vi "update.vi"(8 "error in (no error)":errorcluster, 10 "adapter executability":T1={"instrument"=TRUE, "trajectory"=TRUE, "scanHead"=TRUE, "DAQ"=TRUE, "imageAssembler"=TRUE, "dataCollection"=TRUE, "display"=TRUE, "analyser"=TRUE, "stimulator"=TRUE}, 11 "ImagingModeDL090130Frame in":refnum<class "ImagingModeDL090130Frame.lvclass">=refnum) -> (0 "error out":errorcluster, 3 "ImagingModeDL090130Frame out":refnum<class "ImagingModeDL090130Frame.lvclass">)   [LabVIEW 2010, in "ImagingModeDL090130Frame.lvclass"]
uses:
  ImagingModeDL090130Frame.lvclass
  ImagingModeDL090923Scaffold/ImagingModeDL090923Scaffold/adapter_executability_cluster.ctl
  ImagingModeDL090923Scaffold/ImagingModeDL090923Scaffold/ImagingModeDL090923Scaffold.lvclass
  ScanHead/GenericScanHead/GenericScanHead/GenericScanHead.lvclass
  ImageAssembler/GenericImageAssembler/GenericImageAssembler/GenericImageAssembler.lvclass
  DataCollection/GenericDataCollection/GenericDataCollection/GenericDataCollection.lvclass
  common/xcontrols/XSettings/XSettings/XSettings.xctl
  common/classes/ErrorController/ErrorController/class_data.vi
  common/classes/ErrorController/ErrorController/ErrorController.lvclass
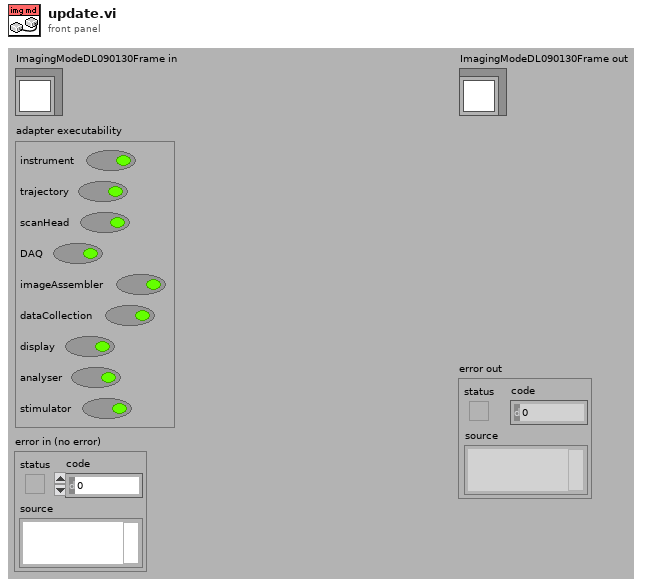
[diagram p1: front panel]
types:
  T1 = typedef "ImagingModeDL090923Scaffold.lvclass/adapter_executability_cluster.ctl" = cluster{"instrument":bool, "trajectory":bool, "scanHead":bool, "DAQ":bool, "imageAssembler":bool, "dataCollection":bool, "display":bool, "analyser":bool, "stimulator":bool}
  T2 = typedef "plugin_specification.ctl" = cluster{"class path":string, "configuration":string, "label":string, "settings name":string}
  T3 = typedef "ImagingModeDL090130Frame.lvclass/control_refs.ctl" = cluster{"resolution controls":cluster{"x pixels":refnum<vi>, "y pixels":refnum<vi>, "ratio x factor":refnum<vi>, "ratio y factor":refnum<vi>, "Vy min(V)":refnum<vi>, "Vy max(V)":refnum<vi>, "Vz min(V)":refnum<vi>, "Vz max(V)":refnum<vi>}, "speed controls":cluster{"pixel dwell time":refnum<vi>, "line scan time":refnum<vi>, "frame rate":refnum<vi>, "keep constant":refnum<vi>}, "number of frames controls":cluster{"# of frames":refnum<vi>, "duration":refnum<vi>, "# of repetitions":refnum<vi>}, "current value indicators":cluster{"frame #":refnum<vi>, "repetition #":refnum<vi>, "offset":refnum<vi>}, "step controls":cluster{"step size":refnum<vi>, "return to origin?":refnum<vi>, "translation mode":refnum<vi>, "XIntensityCompensation":refnum<vi>}, "defineButton":refnum<vi>, "settings enforced?":refnum<vi>, "settings":refnum<vi>}
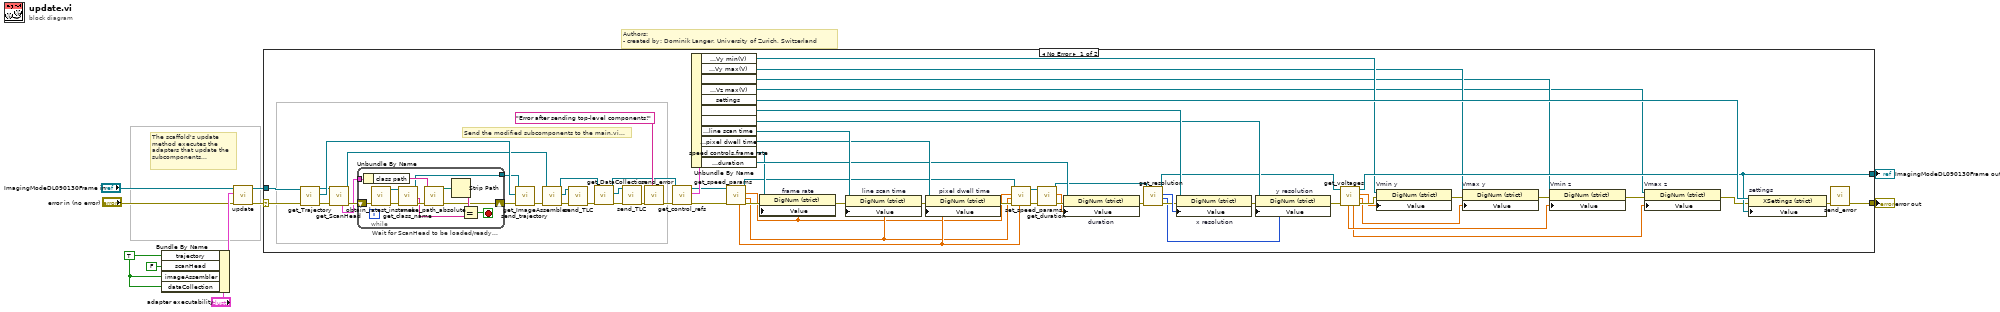
[diagram p0: block diagram]
diagram:
  w3 = TRUE ("instrument")
  # "The scaffold's update method executes the adapters that update the subcomponents..."
  # "Authors: \n- created by: Dominik Langer, University of Zurich, Switzerland"
  n1 = Bundle By Name(cluster="adapter executability", "trajectory"=w3, "scanHead"=FALSE ("instrument"), "imageAssembler"=w3, "dataCollection"=w3) -> (w2:T1)
  n2 = call-parent "update.vi"("error in (no error)"="error in (no error)", "adapter executability"=w2, "ScanModeDL090923Scaffold in"="ImagingModeDL090130Frame in") -> ("error out"=w7:errorcluster, "ScanModeDL090923Scaffold out"=w6:refnum<class "ImagingModeDL090130Frame.lvclass">)  [unwired: 7 in]
  n3 = case shown="No Error" w7 {
    selector: w7 -> [w74 w91]
    tunnel: [w59 w91] -> w10
    tunnel: [w25 w90] -> w9
    tunnel: w6 -> [w73 w90]
    frame No Error {
      # "Send the modified subcomponents to the main.vi..."
      n4 = call-dynamic "get_Trajectory.vi"("error in (no error)"=w74, "ScanModeDL090923Scaffold in"=w73) -> ("error out"=w31:errorcluster, "Trajectory"=w62:refnum<class "GenericTrajectory.lvclass">, "ScanModeDL090923Scaffold out"=w32:refnum<class "ImagingModeDL090130Frame.lvclass">)  [unwired: 2 in, 5 out]
      n5 = call-dynamic "get_ScanHead.vi"("error in (no error)"=w31, "ScanModeDL090923Scaffold in"=w32) -> ("error out"=w30:errorcluster, "ScanModeDL090923Scaffold out"=w29:refnum<class "ImagingModeDL090130Frame.lvclass">, "ScanHead specification"=w28:T2)  [unwired: 4 in, 3 out]
      n6 = while "Wait for ScanHead to be loaded/ready..." {
        shift-right: [w80] -> w63
        shift-left: w30 -> [w89]
        tunnel: w28 -> [w86]
        tunnel: [w78] -> w27
        stop <- w79 stop-if-true
        n7 = Unbundle By Name(w86) -> ("class path"=w85:string)
        n8 = call "obtain_latest_instance.vi"("error in (no error)"=w89) -> ("error out"=w88:errorcluster, "GenericScanHead out"=w87:refnum<class "GenericScanHead.lvclass">)  [unwired: 1 in, 8 out]
        n9 = call-dynamic "get_class_name.vi"("error in (no error)"=w88, "GenericPlugin in"=w87) -> ("error out"=w84:errorcluster, "class file name"=w81:string, "GenericPlugin out"=w78:refnum<class "GenericScanHead.lvclass">)  [unwired: 5 in, 2 out]
        n10 = call "make_path_absolute.vi"("error in (no error)"=w84, "relative path"=w85) -> ("error out"=w80:errorcluster, "absolute path"=w83:path)  [unwired: 8 in]
        n11 = Strip Path(path=w83) -> (name=w82:string)  [unwired: 1 out]
        n12 = Equal?(x=w82, y=w81) -> (x = y?=w79:bool)
      }
      n13 = call-dynamic "send_trajectory.vi"("error in (no error)"=w63, "trajectory"=w62, "GenericScanHead in"=w27) -> ("error out"=w64:errorcluster)  [unwired: 8 out]
      n14 = call-dynamic "get_ImageAssembler.vi"("error in (no error)"=w64, "ScanModeDL090923Scaffold in"=w29) -> ("error out"=w72:errorcluster, "ImageAssembler"=w71:refnum<class "GenericImageAssembler.lvclass">, "ScanModeDL090923Scaffold out"=w67:refnum<class "ImagingModeDL090130Frame.lvclass">)  [unwired: 4 in, 3 out]
      n15 = call-dynamic "send_TLC.vi"("error in (no error)"=w72, "GenericToplevelComponent in"=w71) -> ("error out"=w69:errorcluster)  [unwired: 8 in, 1 out]
      n16 = call-dynamic "get_DataCollection.vi"("error in (no error)"=w69, "ScanModeDL090923Scaffold in"=w67) -> ("error out"=w70:errorcluster, "DataCollection"=w68:refnum<class "GenericDataCollection.lvclass">, "ScanModeDL090923Scaffold out"=w46:refnum<class "ImagingModeDL090130Frame.lvclass">)  [unwired: 4 in, 3 out]
      n17 = call-dynamic "send_TLC.vi"("error in (no error)"=w70, "GenericToplevelComponent in"=w68) -> ("error out"=w60:errorcluster)  [unwired: 8 in, 1 out]
      n18 = call "send_error.vi"("additional message"="Error after sending top-level components!", "error in (no error)"=w60) -> ("error out"=w49:errorcluster)  [unwired: 9 in]
      n19 = call-dynamic "get_control_refs.vi"("error in (no error)"=w49, "ImagingModeDL090130Frame in"=w46) -> ("error out"=w48:errorcluster, "control refs"=w47:T3, "ImagingModeDL090130Frame out"=w45:refnum<class "ImagingModeDL090130Frame.lvclass">)  [unwired: 7 in]
      n20 = Unbundle By Name(w47) -> ("resolution controls.Vy min(V)"=w14:refnum<vi>, "resolution controls.Vy max(V)"=w13:refnum<vi>, "resolution controls.Vz min(V)"=w12:refnum<vi>, "resolution controls.Vz max(V)"=w11:refnum<vi>, "settings"=w34:refnum<vi>, "resolution controls.x pixels"=w43:refnum<vi>, "resolution controls.y pixels"=w42:refnum<vi>, "speed controls.line scan time"=w77:refnum<vi>, "speed controls.pixel dwell time"=w76:refnum<vi>, "speed controls.frame rate"=w57:refnum<vi>, "number of frames controls.duration"=w75:refnum<vi>)
      n21 = call-dynamic "get_speed_params.vi"("error in (no error)"=w48, "ImagingModeDL090130Frame in"=w45) -> ("error out"=w56:errorcluster, "line-scan time"=w36:dbl[unit], "frame rate"=w35:dbl[unit], "ImagingModeDL090130Frame out"=w41:refnum<class "ImagingModeDL090130Frame.lvclass">, "pixel dwell time"=w37:dbl[unit])  [unwired: 4 in, 1 out]
      n22 = property on="frame rate" class="DigNum (strict)"(reference=w57, error in=w56, "Value"=w35) -> (error out=w55:errorcluster)  [unwired: 1 out]
      n23 = property on="line scan time" class="DigNum (strict)"(reference=w77, error in=w55, "Value"=w36) -> (error out=w61:errorcluster)  [unwired: 1 out]
      n24 = property on="pixel dwell time" class="DigNum (strict)"(reference=w76, error in=w61, "Value"=w37) -> (error out=w39:errorcluster)  [unwired: 1 out]
      n25 = call-dynamic "set_speed_params.vi"("pixel-dwell time"=w37, "error in (no error)"=w39, "line-scan time"=w36, "frame rate"=w35, "ImagingModeDL090130Frame in"=w41) -> ("error out"=w38:errorcluster, "ImagingModeDL090130Frame out"=w40:refnum<class "ImagingModeDL090130Frame.lvclass">)  [unwired: 5 in]
      n26 = call-dynamic "get_duration.vi"("error in (no error)"=w38, "ImagingModeDL090130Frame in"=w40) -> ("error out"=w66:errorcluster, "duration"=w65:dbl[unit], "ImagingModeDL090130Frame out"=w44:refnum<class "ImagingModeDL090130Frame.lvclass">)  [unwired: 7 out]
      n27 = property on="duration" class="DigNum (strict)"(reference=w75, error in=w66, "Value"=w65) -> (error out=w54:errorcluster)  [unwired: 1 out]
      n28 = call-dynamic "get_resolution.vi"("error in (no error)"=w54, "ImagingModeDL090130Frame in"=w44) -> ("error out"=w52:errorcluster, "y resolution"=w50:i32, "x resolution"=w53:i32, "ImagingModeDL090130Frame out"=w26:refnum<class "ImagingModeDL090130Frame.lvclass">)  [unwired: 6 in]
      n29 = property on="x resolution" class="DigNum (strict)"(reference=w43, error in=w52, "Value"=w53) -> (error out=w51:errorcluster)  [unwired: 1 out]
      n30 = property on="y resolution" class="DigNum (strict)"(reference=w42, error in=w51, "Value"=w50) -> (error out=w24:errorcluster)  [unwired: 1 out]
      n31 = call-dynamic "get_voltages.vi"("error in (no error)"=w24, "ImagingModeDL090130Frame in"=w26) -> ("error out"=w23:errorcluster, "Vmax_y"=w15:dbl, "Vmin_y"=w18:dbl, "ImagingModeDL090130Frame out"=w25:refnum<class "ImagingModeDL090130Frame.lvclass">, "Vmax_z"=w16:dbl, "Vmin_z"=w17:dbl)  [unwired: 4 in]
      n32 = property on="Vmin y" class="DigNum (strict)"(reference=w14, error in=w23, "Value"=w18) -> (error out=w22:errorcluster)  [unwired: 1 out]
      n33 = property on="Vmax y" class="DigNum (strict)"(reference=w13, error in=w22, "Value"=w15) -> (error out=w21:errorcluster)  [unwired: 1 out]
      n34 = property on="Vmin z" class="DigNum (strict)"(reference=w12, error in=w21, "Value"=w17) -> (error out=w20:errorcluster)  [unwired: 1 out]
      n35 = property on="Vmax z" class="DigNum (strict)"(reference=w11, error in=w20, "Value"=w16) -> (error out=w19:errorcluster)  [unwired: 1 out]
      n36 = property on="settings" class="XSettings (strict)"(reference=w34, error in=w19, "Value"=w25) -> (error out=w33:errorcluster)  [unwired: 1 out]
      n37 = call "send_error.vi"("error in (no error)"=w33) -> ("error out"=w59:errorcluster)  [unwired: 10 in]
    }
    frame Error {
    }
  }
  "error out" <- w10
  "ImagingModeDL090130Frame out" <- w9
